vi "Read Char.vi"(8 "error in (no error)":errorcluster, 11 "ControlKeyDownMsg in":refnum<class "VIKeyDownMsg.lvclass">) -> (0 "error out":errorcluster, 2 "Char":i16, 3 "ControlKeyDownMsg out":refnum<class "VIKeyDownMsg.lvclass">)   [LabVIEW 2018, in "MVA Framework.lvlib" / "ActorEvents.lvlib" / "VIKeyDownMsg.lvclass"]
uses:
  VIKeyDownMsg.lvclass
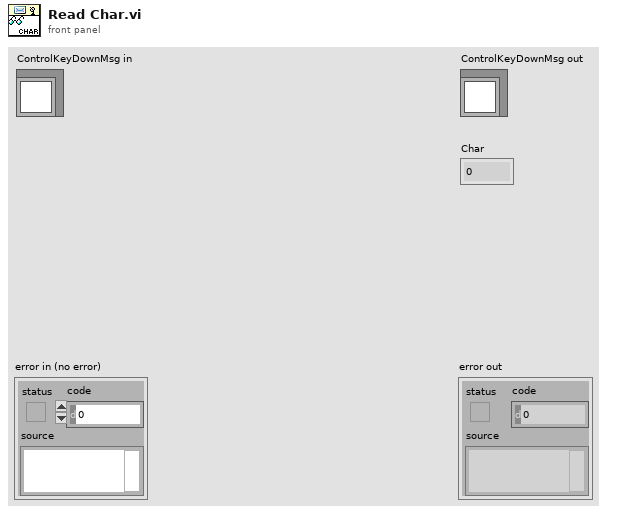
[diagram p1: front panel]
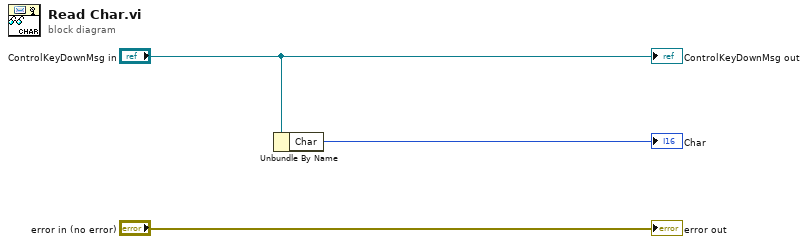
[diagram p0: block diagram]
diagram:
  n1 = Unbundle By Name("ControlKeyDownMsg in") -> ("Char"=→"Char":i16)
  "error out" <- "error in (no error)"
  "ControlKeyDownMsg out" <- "ControlKeyDownMsg in"
